vi "x502_recv_out_cycle.vi"() -> ()   [LabVIEW 2015]
uses:
  <vilib>/Waveform/DWDTOps.llb/DWDT Binary U32 to Digital.vi
panel:
  in  "Частота сигнала (Гц)":dbl=50.0 min=1.0 max=500000.0
  in  "Смещение сигнала":dbl min=-5.0 max=5.0 format="%.2f"
  in  "Амплитуда сигнала":dbl=5.0 min=0.0 max=5.0 format="%.2f"
  in  "Подключение по IP":bool
  in  "IP Addr":string="192.168.0.1"
  out "MCU ver":string
  in  "START":bool
  in  "Список устройств USB/PCIe":u16(ring) items=["E502, 123"]
  out "Mixed Signal Graph":T1(graph)
  in  "Логические каналы":T2(array[cluster])=[{"PhyCh"=1, "Avg"=1, "Mode"=1, "Range"=0}, {"PhyCh"=2, "Avg"=1, "Mode"=1, "Range"=0}, {"PhyCh"=3, "Avg"=1, "Mode"=1, "Range"=0}] {"Range" items=["10 В", "5 В", "2 В", "1 В", "0.5 В", "0.2 В"]; "Mode" items=["С общей землей", "Дифференциальный", "Измерение нуля"]; "Avg" max=255 step=1; "PhyCh" min=1 max=32 step=1}
  in  "Отображать за время":dbl=250.0 min=10.0 step=1.0
  in  "stop":bool
  out "Установленная частота синхронного ввода DIN":dbl=2.0 min=2.0 max=2000000.0 format="%#_8f"
  in  "Частота синхронного ввода DIN":dbl=20000.0 min=1.0 max=2000000.0 format="%#_8f"
  out "FPGA Ver":string
  in  "Количество каналов":u32=3 min=1 max=3
  out "Установленная частота на канал":dbl=2.0 min=2.0 max=2000000.0 format="%#_8f"
  out "Установленная частота сбора":dbl=2.0 min=2.0 max=2000000.0 format="%#_8f"
  in  "Частота сбора на канал":dbl=2000000.0 min=2.0 max=2000000.0 format="%#_8f"
  in  "Частота сбора (Гц)":dbl=2000000.0 min=2.0 max=2000000.0 format="%#_8f"
  out "PldaVer":u8
  out "Serial":string
  out "Name":string
  # "Информация о плате"
  # "Настройки модуля"
  # "Устанавливаемое"
  # "Установленное"
  # "Вывод на ЦАП"
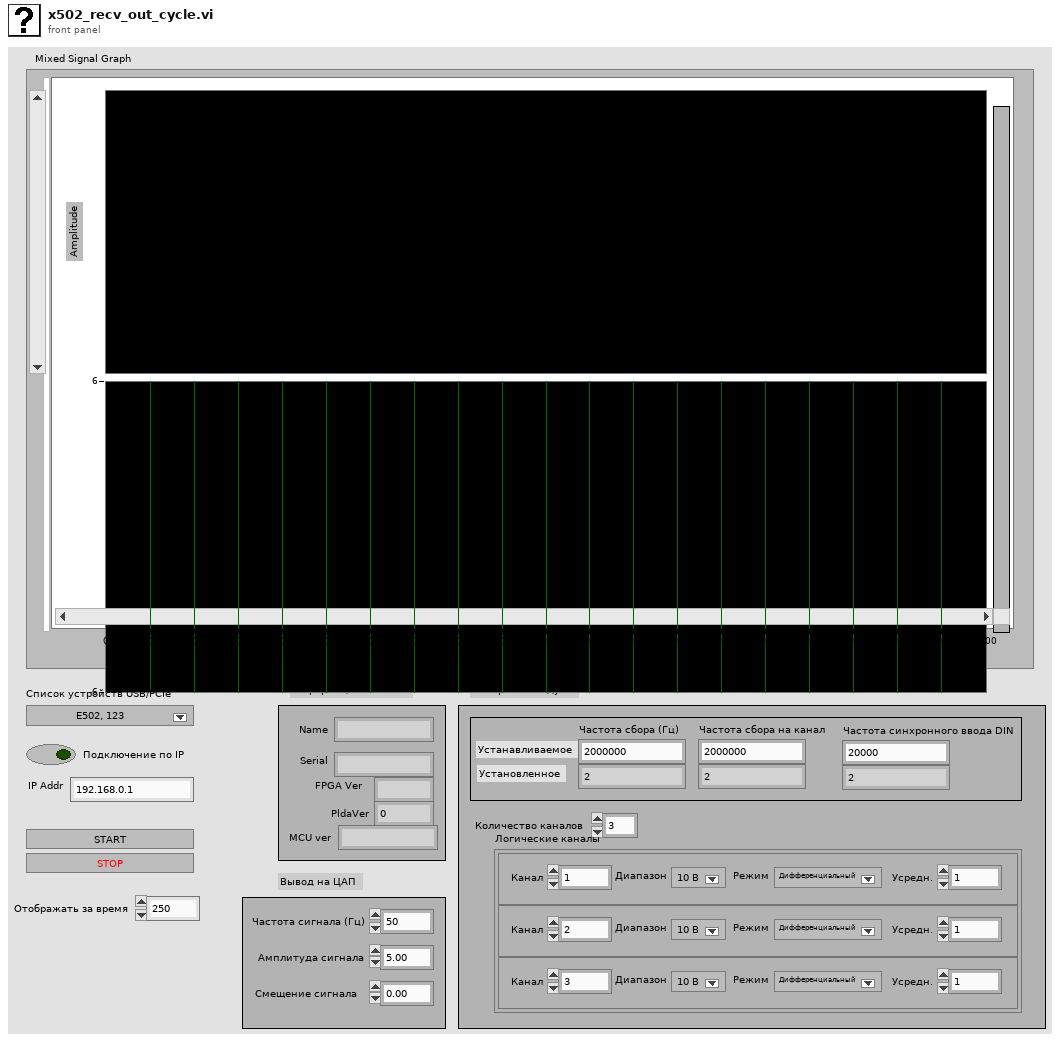
[diagram p1: front panel]
types:
  T1 = cluster{"Dynamic Data Type":dynamicdata, "digital waveform":digitalwaveform}
  T2 = cluster{"PhyCh":u32, "Avg":u32, "Mode":u32, "Range":u32}[]
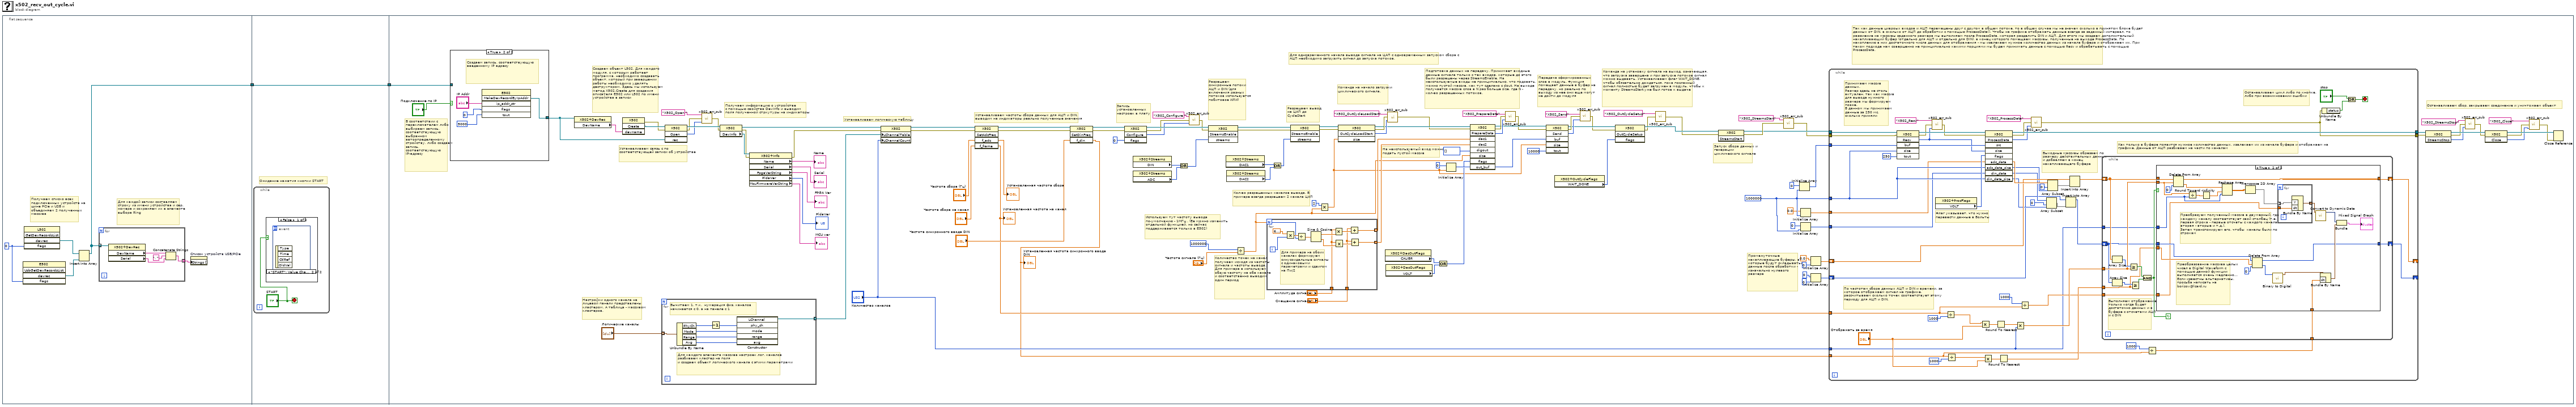
[diagram p0: block diagram]
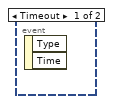
[diagram p2: hidden frame]
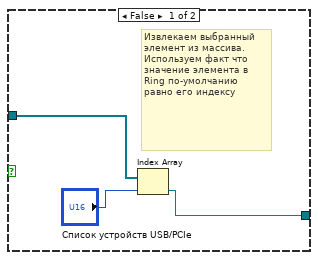
[diagram p5: hidden frame]
diagram:
  n1 = flat-sequence {
    tunnel: [w3] -> w1
    tunnel: [w13] -> w2
    tunnel: w1 -> [w13]
    tunnel: w2 -> [w93]
    frame #0 {
      w5 = 0
      # "Для каждой записи составляем строку из имени устройства и сер. номера и сохраняем их в элементе выбора Ring"
      # "Получаем списко всех подключенных устройств на шине PCIe и USB и объединяем 2 полученных массива"
      n2 = invoke class="E502" method="UsbGetDevRecordsList"("flags"=w5) -> ("devrec"=w6:refnum<k24>[])  [unwired: 4 in, 4 out]
      n3 = invoke class="L502" method="GetDevRecordsList"("flags"=w5) -> ("devrec"=w7:refnum<k24>[])  [unwired: 4 in, 4 out]
      n4 = Insert Into Array(array=w7, new element=w6) -> (w3:refnum<k24>[])  [unwired: 1 in]
      n5 = for {
        tunnel: [w9] -> w4 mode=indexing
        tunnel: w3 -> [w8] mode=indexing
        n6 = property class="X502+DevRec"(reference=w8) -> ("DevName"=w12:string, "Serial"=w10:string)  [unwired: 1 in, 2 out]
        n7 = Concatenate Strings(w12, ", ", w10) -> (w9:string)
      }
      n8 = property on="Список устройств USB/PCIe" class="Ring (strict)"("Strings []"=w4) -> ()  [unwired: 2 in, 2 out]
    }
    frame #1 {
      # "Ожидание нажатия кнопки START"
      n9 = while {
        stop <- "START" stop-if-true
        n10 = case shown="False" "START" {
          frame False {
            n11 = event shown="[1] \"START\": Value Change" {
              selector: _ -> [_ _]
              dyn-events: _ -> [_ _]
              timeout: _ -> [_ _]
              event Timeout {
                n12 = event-data() -> ()  [unwired: 1 in, 2 out]
              }
              event "START": Value Change {
                n13 = event-data() -> ()  [unwired: 1 in, 4 out]
              }
            }
          }
          frame True {
          }
        }
      }
    }
    frame #2 {
      w85 = u32 1000000 ("element")
      # "Команда на установку сигнала на выход, означающая, что загрузка завершена и при запуске потоков сигнал можно выдавать. Устанавливаем флаг WAIT_DONE, чтобы обязательно дождаться, пока посланный сигнал полностью будет загружен в модуль, чтобы к моменту StreamsStart уже был готов к выдаче"
      # "Передача сформированных слов в модуль. Функция помещает данные в буфер на передачу, но раельно по выходу из нее они еще могут не дойти до модуля"
      # "Подготовка данных на передачу. Принимает входные данные сигнала только с тех входов, которые до этого были разрешены через StreamsEnable. На неиспользуемые входы не принципиально, что подовать, можно пустой массив, как тут сделано с dout. На выходе получается массив слов в N раз больше size, где N - кол-во разрешенных потоков."
      # "Команда на начало загрузки циклического сигнала."
      # "Для одновременного начала вывода сигнала на ЦАП с одновременным запуском сбора с АЦП необходимо загрузить сигнал до запуска потоков."
      # "На неиспользуемый вход можно подать пустой массив"
      # "Кол-во разрешенных каналов вывода. В примере всегда разрешаем 2 канала ЦАП"
      # "Количество точек на канал получаем исходя из частоты сигнала и частоты вывода. Для примера в используем обзую частоту на оба канала и соответственно выводим один период"
      # "Используем тут частоту вывода по-умолчанию - 1МГц . (Ее можно изменить отдельной функцией, но сейчас поддерживается только в E502)"
      # "Разрешаем вывод на ЦАП до CycleStart"
      # "Останавливаем сбор, закрываем соединение и уничтожаем объект"
      # "Так как данные цивроых входов и АЦП перемешены друг с другом в общем потоке, то в общем случае мы не значем сколько в принятом блоке будет данных от DIN, а сколько от АЦП до обработки с помощью ProcessData(). Чтобы на графике отображать данные всегда за заданный интервал, то разюиение на массивы заданного размера мы выполняем после ProcessData, которая разделить DIN и АЦП. Для этого мы создаем дополнительный накапливающий буфер (отдельно для АЦП и отдельно для DIN), в конец которого помещаем массивы, полученные на выходе ProcessData. По накоплению в них достаточного числа данных для отображения - мы извлекаем нужное количество данных из начала буфера и отображаем их. При таком подходе нам совершенно не принципиально какими порциями мы будем принимать данные с помощью Recv и обрабатывать с помощью ProcessData."
      # "Промежуточные накапливающие буферы, в которые будут складываться данные после обработки - изначально нулевого размера"
      # "Запуск сбора данных и генерации циклического сигнала"
      # "Разрешаем синхронные потоки АЦП и DIN (для включения разных потоков используется побитовое ИЛИ)"
      # "В соответствии с переключателем либо выбираем запись, соответствующую выбранном автоопределенному стройству, либо создаем запись, соответствующую IP-адресу"
      # "Запись установленных настроек в плату"
      # "Устанавливаем частоты сбора данных для АЦП и DIN,\nвыводим на индикаторы реально полученные значения"
      # "Устанавливаем логическую таблицу"
      # "Настройки одного канала на лицевой панели представлены кластером. А таблица - массивом кластеров."
      # "Создаем объект L502. Для каждого модуля, с которым работает программа, необходимо создавать объект, который при завершении работы необходимо удалять деструктором. Здесь мы используем метод X502.Create для создания описателя E502 или L502 по имени устройства в записи"
      # "Получаем информацию о устройстве \nс помощью свойства DevInfo и выводим\nполя полученной стркутуры на индикаторы"
      # "Устанавливаем связь с по соответствующей записи об устройстве"
      n14 = case shown="True" "Подключение по IP" {
        tunnel: w93 -> [w241 _]
        tunnel: [w239 w242] -> w92
        frame False {
          # "Извлекаем выбранный элемент из массива. Используем факт что значение элемента в Ring по-умолчанию равно его индексу"
          n15 = Index Array(array=w241, index="Список устройств USB/PCIe") -> (element=w239:refnum<k24>)
        }
        frame True {
          # "Создаем запись, соответствующую введенному IP адресу"
          n16 = invoke class="E502" method="MakeDevRecordByIpAddr"("ip_addr_str"="IP Addr", "flags"=0, "tout"=5000) -> ("MakeDevRecordByIpAddr"=w242:refnum<k24>)  [unwired: 3 in, 5 out]
        }
      }
      n17 = property class="X502+DevRec"(reference=w92) -> ("DevName"=w113:string)  [unwired: 1 in, 2 out]
      n18 = invoke class="X502" method="Create"("devname"=w113) -> (error out=w112:errorcluster, "Create"=w114:refnum<k24>)  [unwired: 3 in, 2 out]
      n19 = for {
        tunnel: "Логические каналы" -> [w252] mode=indexing
        tunnel: [w246] -> w130 mode=indexing
        # "Вычитаем 1, т.к.  нумерация физ. каналов начинается с 0, а на панеле с 1"
        # "Для каждого элемента массива настроек лог. каналов разбиваем кластер на поля\nи создаем объект логического канала с этими параметрами"
        n20 = Unbundle By Name(w252) -> ("PhyCh"=w251:u32, "Mode"=w249:u32, "Range"=w248:u32, "Avg"=w247:u32)
        n21 = Decrement(x=w251) -> (x-1=w250:u32)
        n22 = constructor class="X502+LChannel"("phy_ch"=w250, "mode"=w249, "range"=w248, "avg"=w247) -> (reference out=w246:refnum<k24>)  [unwired: 3 in, 6 out]
      }
      n23 = invoke class="X502" method="Open"(reference=w114, error in=w112, "rec"=w92) -> (reference out=w115:refnum<k24>, error out=w110:errorcluster, "Open"=w111:i32)  [unwired: 1 in, 1 out]
      n24 = call "x502_err_sub.vi"("Error code"=w111, "error in (no error)"=w110, "Error descr"="X502_Open ") -> ("error out"=w108:errorcluster)
      n25 = property class="X502"(reference=w115, error in=w108) -> (reference out=w116:refnum<k24>, error out=w106:errorcluster, "DevInfo"=w107:refnum<k24>)
      n26 = property class="X502+Info"(reference=w107, error in=w106) -> (error out=w94:errorcluster, "Name"=→"Name":string, "Serial"=→"Serial":string, "FpgaVerString"=→"FPGA Ver":string, "PldaVer"=→"PldaVer":u8, "McuFirmwareVerString"=→"MCU ver":string)  [unwired: 1 out]
      n27 = property class="X502"(reference=w116, error in=w94, "LChannelTable"=w130, "LChannelCount"="Количество каналов") -> (reference out=w117:refnum<k24>, error out=w118:errorcluster)
      n28 = invoke class="X502" method="SetAdcFreq"(reference=w117, error in=w118, "f_adc"="Частота сбора (Гц)", "f_frame"="Частота сбора на канал") -> (reference out=w122:refnum<k24>, error out=w123:errorcluster, "f_adc"=→"Установленная частота сбора":dbl, "f_frame"=w61:dbl)  [unwired: 1 in, 1 out]
      "Установленная частота на канал" <- w61
      n29 = invoke class="X502" method="SetDinFreq"(reference=w122, error in=w123, "f_din"="Частота синхронного ввода DIN") -> (reference out=w127:refnum<k24>, error out=w128:errorcluster, "f_din"=w59:dbl)  [unwired: 1 in, 1 out]
      "Установленная частота синхронного ввода DIN" <- w59
      n30 = invoke class="X502" method="Configure"(reference=w127, error in=w128, "flags"=0) -> (reference out=w129:refnum<k24>, error out=w100:errorcluster, "Configure"=w98:i32)  [unwired: 1 in, 1 out]
      n31 = property class="X502+Streams"() -> ("DIN"=w96:u32)  [unwired: 2 in, 2 out]
      n32 = property class="X502+Streams"() -> ("ADC"=w126:u32)  [unwired: 2 in, 2 out]
      n33 = Or(x=w96, y=w126) -> (x .or. y?=w95:u32)
      n34 = call "x502_err_sub.vi"("Error code"=w98, "error in (no error)"=w100, "Error descr"="X502_Configure ") -> ("error out"=w99:errorcluster)
      n35 = invoke class="X502" method="StreamsEnable"(reference=w129, error in=w99, "streams"=w95) -> (reference out=w53:refnum<k24>, error out=w52:errorcluster)  [unwired: 1 in, 2 out]
      n36 = property class="X502+Streams"() -> ("DAC1"=w55:u32)  [unwired: 2 in, 2 out]
      n37 = property class="X502+Streams"() -> ("DAC2"=w56:u32)  [unwired: 2 in, 2 out]
      n38 = Divide(x=1000000, y="Частота сигнала (Гц)") -> (x/y=w40:dbl)
      n39 = for {
        N: w40 -> [w141]
        tunnel: [w135] -> w44 mode=indexing
        tunnel: [w134] -> w43 mode=indexing
        tunnel: "Амплитуда сигнала" -> [w133]
        tunnel: "Смещение сигнала" -> [w132]
        i -> [w143]
        # "Для примера на обоих каналах формируем синусоидальные сигналы с одинаковыми параметрами и сдвигом на Пи/2"
        n40 = Multiply(x=6.283185307179586, y=w143) -> (x*y=w142:dbl)
        n41 = Divide(x=w142, y=w141) -> (x/y=w140:dbl)
        n42 = Sine & Cosine(0:w140) -> (1:w139:dbl, 2:w137:dbl)
        n43 = Multiply(x=w133, y=w139) -> (x*y=w138:dbl)
        n44 = Multiply(x=w133, y=w137) -> (x*y=w136:dbl)
        n45 = Add(x=w132, y=w138) -> (x+y=w135:dbl)
        n46 = Add(x=w132, y=w136) -> (x+y=w134:dbl)
      }
      n47 = Or(x=w55, y=w56) -> (x .or. y?=w54:u32)
      n48 = invoke class="X502" method="StreamsEnable"(reference=w53, error in=w52, "streams"=w54) -> (reference out=w51:refnum<k24>, error out=w50:errorcluster)  [unwired: 1 in, 2 out]
      n49 = Multiply(x=2, y=w40) -> (x*y=w29:dbl)
      n50 = invoke class="X502" method="OutCycleLoadStart"(reference=w51, error in=w50, "size"=w29) -> (reference out=w45:refnum<k24>, error out=w47:errorcluster, "OutCycleLoadStart"=w48:i32)  [unwired: 1 in, 1 out]
      n51 = property class="X502+DacOutFlags"() -> ("CALIBR"=w37:u32)  [unwired: 2 in, 2 out]
      n52 = property class="X502+DacOutFlags"() -> ("VOLT"=w36:u32)  [unwired: 2 in, 2 out]
      n53 = call "x502_err_sub.vi"("Error code"=w48, "error in (no error)"=w47, "Error descr"="X502_OutCycleLoadStart") -> ("error out"=w42:errorcluster)
      n54 = Or(x=w37, y=w36) -> (x .or. y?=w35:u32)
      n55 = Initialize Array(u32 0 ("element"), w29) -> (w38:u32[])
      n56 = invoke class="X502" method="PrepareData"(reference=w45, error in=w42, "dac1"=w44, "dac2"=w43, "digout"=i32[] [], "size"=w40, "flags"=w35, "out_buf"=w38) -> (reference out=w31:refnum<k24>, error out=w32:errorcluster, "PrepareData"=w33:i32, "out_buf"=w30:u32[])  [unwired: 1 in, 5 out]
      n57 = call "x502_err_sub.vi"("Error code"=w33, "error in (no error)"=w32, "Error descr"="X502_PrepareData") -> ("error out"=w27:errorcluster)
      n58 = invoke class="X502" method="Send"(reference=w31, error in=w27, "buf"=w30, "size"=w29, "tout"=u32 10000 ("element")) -> (reference out=w23:refnum<k24>, error out=w24:errorcluster, "Send"=w25:i32)  [unwired: 1 in, 3 out]
      n59 = property class="X502+OutCycleFlags"() -> ("WAIT_DONE"=w15:u32)  [unwired: 2 in, 2 out]
      n60 = call "x502_err_sub.vi"("Error code"=w25, "error in (no error)"=w24, "Error descr"="X502_Send") -> ("error out"=w22:errorcluster)
      n61 = invoke class="X502" method="OutCycleSetup"(reference=w23, error in=w22, "flags"=w15) -> (reference out=w21:refnum<k24>, error out=w19:errorcluster)  [unwired: 1 in, 2 out]
      n62 = call "x502_err_sub.vi"("error in (no error)"=w19, "Error descr"="X502_OutCycleSetup") -> ("error out"=w18:errorcluster)  [unwired: 1 in]
      n63 = invoke class="X502" method="StreamsStart"(reference=w21, error in=w18) -> (reference out=w73:refnum<k24>, error out=w75:errorcluster)  [unwired: 1 in, 1 out]
      n64 = call "x502_err_sub.vi"("error in (no error)"=w75, "Error descr"="X502_StreamsStart") -> ("error out"=w72:errorcluster)  [unwired: 1 in]
      n65 = Initialize Array(u32 0 ("element"), w85) -> (w86:u32[])
      n66 = Initialize Array(0.0 ("element"), w85) -> (w88:dbl[])
      n67 = Initialize Array(u32 0 ("element"), w85) -> (w87:u32[])
      n68 = Initialize Array(0.0 ("element"), u32 0 ("element")) -> (w90:dbl[])
      n69 = Initialize Array(u32 0 ("element"), u32 0 ("element")) -> (w89:u32[])
      n70 = while {
        tunnel: w73 -> [w197]
        tunnel: w72 -> [w196]
        tunnel: [w195] -> w71
        tunnel: w86 -> [w194]
        shift-right: [w189] -> _
        shift-left: w90 -> [w188]
        shift-right: [w160] -> _
        shift-left: w89 -> [w178]
        tunnel: "Количество каналов" -> [w145]
        tunnel: w61 -> [w161]
        tunnel: w59 -> [w163]
        tunnel: w85 -> [w159]
        tunnel: w87 -> [w158]
        tunnel: w88 -> [w157]
        tunnel: [w146] -> w70
        stop <- w166 stop-if-true
        # "Останавливаем цикл либо по кнопке, либо при возникновении ошибки"
        # "Как только в буфере появится нужное количество данных, извлекаем их из начала буфера и отображаем на графике. Данные от АЦП разбиваем на части по каналам"
        # "По частотам сбора данных АЦП и DIN и времени, за которое отображаем сигнал на графике, рассчитываем сколько точек соответствует этому периоду для АЦП и DIN."
        # "Выходные массивы обрезаем по размеру действительных данных и добавляем в конец накапливающего буфера"
        # "Флаг указывает, что нужно перевести данные в Вольты"
        # "Принимаем массив данных.\nРазмер здесь не столь актуален, так как массив для вывода нужного размера мы формируем позже.\nВ данном мы принимаем данные за 250 мс, сколько приняли"
        n71 = invoke class="X502" method="Recv"(reference=w197, error in=w196, "buf"=w194, "size"=w159, "tout"=u32 250 ("element")) -> (reference out=w185:refnum<k24>, error out=w153:errorcluster, "Recv"=w152:i32, "buf"=w193:u32[])  [unwired: 1 in, 2 out]
        n72 = call "x502_err_sub.vi"("Error code"=w152, "error in (no error)"=w153, "Error descr"="X502_Recv") -> ("error out"=w151:errorcluster)
        n73 = property class="X502+ProcFlags"() -> ("VOLT"=w184:u32)  [unwired: 2 in, 2 out]
        n74 = Divide(x=w161, y=1000) -> (x/y=w176:dbl)
        n75 = Divide(x=w163, y=1000) -> (x/y=w172:dbl)
        n76 = Multiply(x=w176, y="Отображать за время") -> (x*y=w175:dbl)
        n77 = Multiply(x=w172, y="Отображать за время") -> (x*y=w171:dbl)
        n78 = invoke class="X502" method="ProcessData"(reference=w185, error in=w151, "src"=w193, "size"=w152, "flags"=w184, "adc_data"=w157, "adc_data_size"=w159, "din_data"=w158, "din_data_size"=w159) -> (reference out=w195:refnum<k24>, error out=w149:errorcluster, "ProcessData"=w148:i32, "adc_data"=w191:dbl[], "adc_data_size"=w186:u32, "din_data"=w181:u32[], "din_data_size"=w180:u32)  [unwired: 1 in, 3 out]
        n79 = Round To Nearest(number=w175) -> (nearest integer value=w174:dbl)
        n80 = Round To Nearest(number=w171) -> (nearest integer value=w167:dbl)
        n81 = Multiply(x=w174, y=w145) -> (x*y=w168:dbl)
        n82 = Divide(x=u32 1000 ("element"), y=w161) -> (x/y=w156:dbl)
        n83 = call "x502_err_sub.vi"("Error code"=w148, "error in (no error)"=w149, "Error descr"="X502_ProcessData") -> ("error out"=w146:errorcluster)
        n84 = Array Subset(array=w181, index=u32 0 ("element"), length=w180) -> (w179:u32[])
        n85 = Array Subset(array=w191, index=u32 0 ("element"), length=w186) -> (w183:dbl[])
        n86 = Insert Into Array(array=w178, new element=w179) -> (w169:u32[])  [unwired: 1 in]
        n87 = Insert Into Array(array=w188, new element=w183) -> (w187:dbl[])  [unwired: 1 in]
        n88 = Divide(x=u32 1000 ("element"), y=w163) -> (x/y=w155:dbl)
        n89 = while {
          shift-right: [w211] -> w189
          shift-left: w187 -> [w210]
          shift-right: [w201] -> w160
          shift-left: w169 -> [w203]
          tunnel: w168 -> [w208]
          tunnel: w167 -> [w202]
          tunnel: w156 -> [w200]
          tunnel: w155 -> [w199]
          tunnel: w145 -> [w198]
          stop <- w204 continue-if-true
          # "Выполняем отображение только когда будет достаточно данных и в буфере с отсчетами АЦП и с DIN"
          n90 = Array Size(array=w203) -> (size(s)=w207:i32)
          n91 = Array Size(array=w210) -> (size(s)=w209:i32)
          n92 = Greater Or Equal?(x=w209, y=w208) -> (x >= y?=w205:bool)
          n93 = Greater Or Equal?(x=w207, y=w202) -> (x >= y?=w206:bool)
          n94 = And(x=w205, y=w206) -> (x .and. y?=w204:bool)
          n95 = case shown="True" w204 {
            tunnel: [w213 w235] -> w211
            tunnel: w210 -> [w213 w234]
            tunnel: w208 -> [_ w219]
            tunnel: w203 -> [w212 w225]
            tunnel: w202 -> [_ w224]
            tunnel: [w212 w229] -> w201
            tunnel: w200 -> [_ w217]
            tunnel: w199 -> [_ w227]
            tunnel: w198 -> [_ w214]
            frame False {
            }
            frame True {
              # "Преобразуем полученный массив в двумерный, где каждому каналу соответствует свой столбец (т.е. первая строка - первые отсчеты с каждого канала, вторая - вторые и т.д.).\nЗатем транспонируем его, чтобы  каналы были по строкам"
              # "Преобразование массива целых чисел в Digital Waveform с помощью данной функции выполняется очень медленно... Если известны альтернативы, просьба написать на borisov@lcard.ru"
              n96 = Delete From Array(array=w234, length=w219, index=u32 0 ("element")) -> (deleted portion=w218:dbl[], array with subset deleted=w235:dbl[])
              n97 = Divide(x=w219, y=w214) -> (x/y=w223:dbl)
              n98 = Round Toward -Infinity(1:w223) -> (0:w220:dbl)
              n99 = Reshape Array(w218, w220, w214) -> (w222:dbl[][])
              n100 = Transpose 2D Array(2D array=w222) -> (transposed array=w221:dbl[][])
              n101 = Delete From Array(array=w225, length=w224, index=u32 0 ("element")) -> (deleted portion=w231:u32[], array with subset deleted=w229:u32[])
              n102 = call-poly <vilib>:"Binary to Digital.vi"("binary array"=w231) -> ("digital waveform"=w226:digitalwaveform)  [unwired: 9 in, 1 out]
              n103 = for {
                tunnel: w221 -> [w237] mode=indexing
                tunnel: w217 -> [w238]
                tunnel: [w236] -> w216 mode=indexing
                n104 = Bundle By Name("Y"=w237, "dt"=w238) -> (w236:waveform(dbl))  [unwired: 1 in]
              }
              n105 = call "Convert to Dynamic Data"("Array of Waveforms"=w216) -> ("Dynamic Data Type"=w215:dynamicdata)  [unwired: 3 out]
              n106 = Bundle By Name(cluster=w226, "dt"=w227) -> (w230:digitalwaveform)
              n107 = Bundle("Dynamic Data Type"=w215, "digital waveform"=w230) -> (→"Mixed Signal Graph":T1)  [unwired: 1 in]
            }
          }
        }
        n108 = Unbundle By Name(w146) -> ("status"=w147:bool)
        n109 = Or(x="stop", y=w147) -> (x .or. y?=w166:bool)
      }
      n110 = invoke class="X502" method="StreamsStop"(reference=w71, error in=w70) -> (reference out=w76:refnum<k24>, error out=w69:errorcluster, "StreamsStop"=w67:i32)  [unwired: 1 in]
      n111 = call "x502_err_sub.vi"("Error code"=w67, "error in (no error)"=w69, "Error descr"="X502_StreamsStop") -> ("error out"=w66:errorcluster)
      n112 = invoke class="X502" method="Close"(reference=w76, error in=w66) -> (reference out=w77:refnum<k24>, error out=w64:errorcluster, "Close"=w63:i32)  [unwired: 1 in]
      n113 = call "x502_err_sub.vi"("Error code"=w63, "error in (no error)"=w64, "Error descr"="X502_Close") -> ("error out"=w62:errorcluster)
      n114 = Close Reference(reference=w77, error in (no error)=w62) -> ()  [unwired: 1 out]
    }
  }
